vi "testNumeric.vi"(8 "error in (no error)":errorcluster, 11 "TestCase in":refnum<class "Test Status Updater.lvclass">) -> (0 "error out":errorcluster, 3 "TestCase out":refnum<class "Test Status Updater.lvclass">)   [LabVIEW 2014, in "Test Status Updater.lvclass"]
uses:
  Test Status Updater.lvclass
  Test Status Updater.lvclass/Test Status Updater.ctl
  Core/Shared/Classes/Status Updater/Status Updater.lvclass/Status Updater.ctl
  Core/Shared/Classes/Status Events/Create.vi
  <vilib>/addons/_JKI Toolkits/VI Tester/TestCase.llb/TestCase.lvclass
  Core/Shared/Classes/Status Events/Status Events.lvclass
  Core/Shared/Classes/Status Updater/Status Updater.lvclass
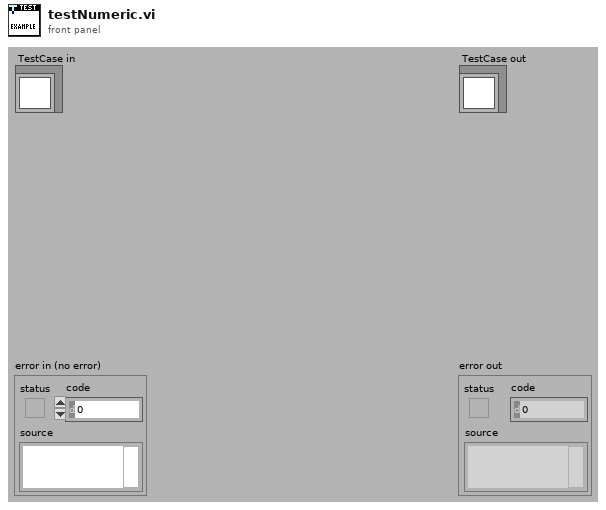
[diagram p1: front panel]
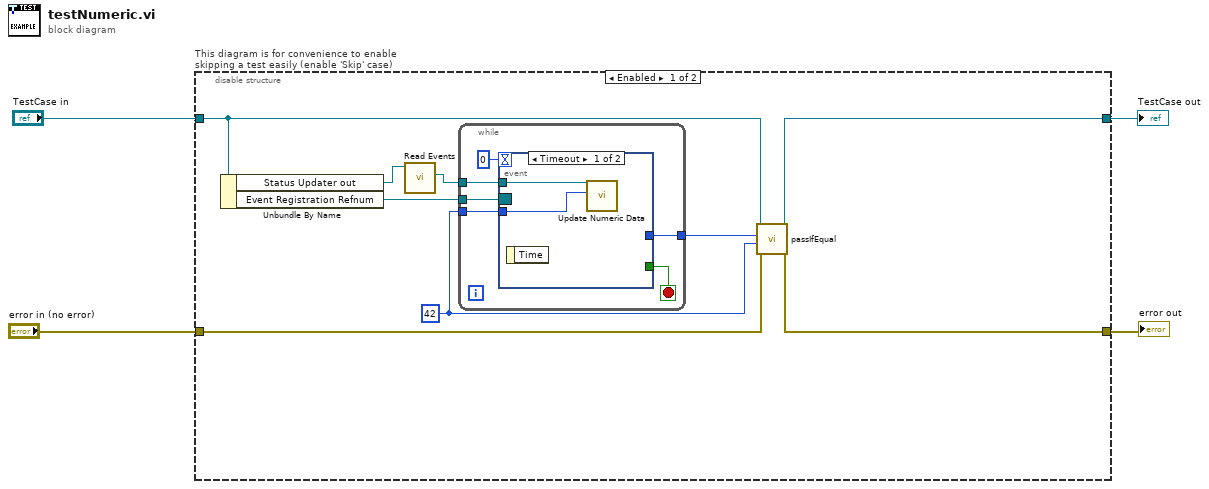
[diagram p0: block diagram]
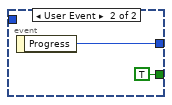
[diagram p2: hidden frame]
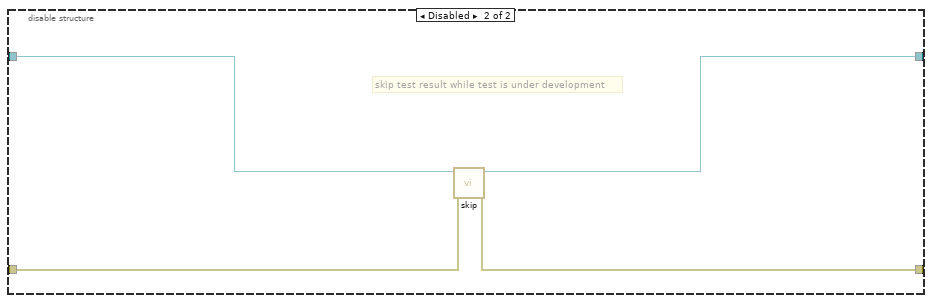
[diagram p3: hidden frame]
diagram:
  n1 = disable-structure "This diagram is for convenience to enable skipping a test easily (enable 'Skip' case)" shown="Enabled" {
    disable-tunnel: "TestCase in" -> [w8 w27]
    disable-tunnel: [w13 w25] -> w1
    disable-tunnel: [w12 w26] -> w3
    disable-tunnel: "error in (no error)" -> [w11 w24]
    frame Enabled {
      w5 = u32 42 ("Numeric Data")
      n2 = Unbundle By Name(w8) -> ("Status Updater out"=w9:refnum<class "Status Updater.lvclass">, "Event Registration Refnum"=w10:refnum<event-registration>)
      n3 = call "Read Events.vi"("Status Updater in"=w9) -> ("Status Events"=w7:refnum<class "Status Events.lvclass">)  [unwired: 10 in]
      n4 = while {
        tunnel: w10 -> [w18]
        tunnel: [w17] -> w6
        tunnel: w7 -> [w16]
        tunnel: w5 -> [w15]
        stop <- w14 stop-if-true
        n5 = event shown="[0] Timeout" {
          selector: w18 -> [_ _]
          dyn-events: _ -> [_ _]
          timeout: 0 -> [_ _]
          tunnel: w16 -> [w21 _]
          tunnel: [_ w23] -> w17
          tunnel: w15 -> [w20 _]
          tunnel: [_ TRUE] -> w14
          event Timeout {
            n6 = event-data() -> ()  [unwired: 1 in, 1 out]
            n7 = call "Update Numeric Data.vi"("Numeric Data"=w20, "Status Updater in"=w21) -> ()  [unwired: 8 in, 2 out]
          }
          event User Event {
            n8 = event-data() -> ("Progress"=w23:u32)  [unwired: 1 in]
          }
        }
      }
      n9 = call-dynamic "passIfEqual.vi"("error in (no error)"=w11, "y"=w5, "x"=w6, "TestCase in"=w8) -> ("error out"=w12:errorcluster, "TestCase out"=w13:refnum<class "Test Status Updater.lvclass">)  [unwired: 6 in]
    }
    frame Disabled {
      # "skip test result while test is under development"
      n10 = call <vilib>:"skip.vi"("error in (no error)"=w24, "TestCase in"=w27) -> ("error out"=w26:errorcluster, "TestCase out"=w25:refnum<class "Test Status Updater.lvclass">)  [unwired: 8 in]
    }
  }
  "error out" <- w3
  "TestCase out" <- w1
